vi "Initialize.vi"(8 "error in (no error)":errorcluster, 11 "UDPlog Transfer Rx User Interface in":refnum<class "UDPlog Transfer Rx User Interface.lvclass">) -> (0 "error out":errorcluster, 3 "UDPlog Transfer Rx User Interface out":refnum<class "UDPlog Transfer Rx User Interface.lvclass">)   [LabVIEW 2023, in "UDPlog.lvlib" / "UDPlog Transfer Rx User Interface.lvclass"]
uses:
  UDPlog Transfer Rx User Interface.lvclass
  C:/Users/Public/Documents/National Instruments/NI VeriStand 2023/Custom Devices/Data Sharing Framework/Linux_x64/DSF Core.lvlibp/Classes/User Interface/User Interface.lvclass
  Configurations/Rx Transfer/UDPlog Transfer Rx Configuration.lvclass
  C:/Users/Public/Documents/National Instruments/NI VeriStand 2023/Custom Devices/Data Sharing Framework/Linux_x64/DSF Core.lvlibp/Classes/Configuration/Configuration.lvclass
  Users/Public/Documents/National Instruments/NI VeriStand 2023/Custom Devices/Data Sharing Framework/Linux_x64/DSF Core.lvlibp/Classes/User Interface/User Interface.lvclass
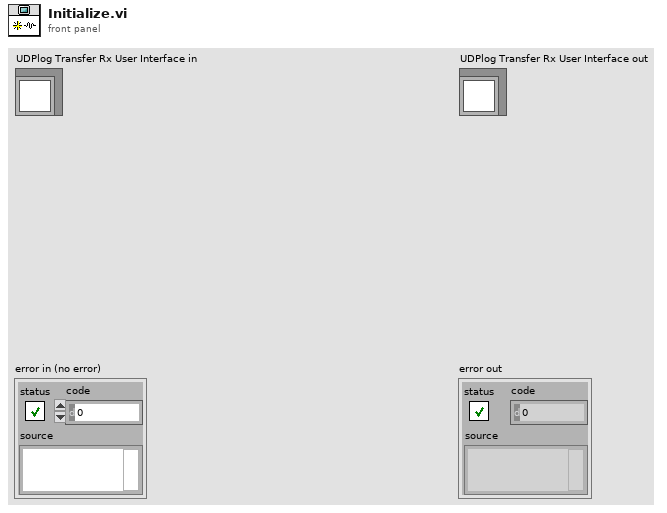
[diagram p1: front panel]
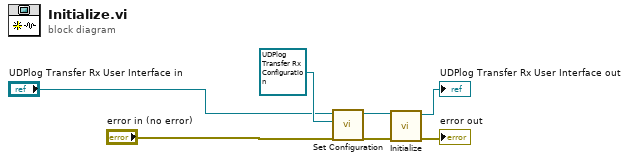
[diagram p0: block diagram]
diagram:
  n1 = call "Set Configuration.vi"("configuration"=refnum<class "UDPlog Transfer Rx Configuration.lvclass"> refnum ("UDPlog.lvlib:UDPlog Transfer Rx Configuration.lvclass"), "User Interface in"="UDPlog Transfer Rx User Interface in") -> ("User Interface out"=w3:refnum<class "UDPlog Transfer Rx User Interface.lvclass">)  [unwired: 8 in, 1 out]
  n2 = call-parent "Initialize.vi"("error in (no error)"="error in (no error)", "User Interface in"=w3) -> ("error out"=→"error out":errorcluster, "User Interface out"=→"UDPlog Transfer Rx User Interface out":refnum<class "UDPlog Transfer Rx User Interface.lvclass">)  [unwired: 8 in]
